vi "DaxKeyboardControl.vi"(8 "PlatMods":T1, 10 "Char":i16, 11 "Daxsonics Settings":refnum<vi>) -> ()   [LabVIEW 2022 SP3]
uses:
  Dax_Control_Cluster.ctl
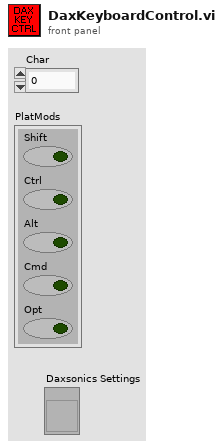
[diagram p1: front panel]
types:
  T1 = cluster{"Shift":bool, "Ctrl":bool, "Alt":bool, "Cmd":bool, "Opt":bool}
  T2 = typedef "Dax_Control_Cluster.ctl" = cluster{"Freq (MHz) ":u16, "Voltage (V)":u16, "Gain (dB)":u16}
  T3 = typedef "LVStringsAndValuesArrayTypeDef_U16.ctl" = cluster{"String":string, "Value":u16}[]
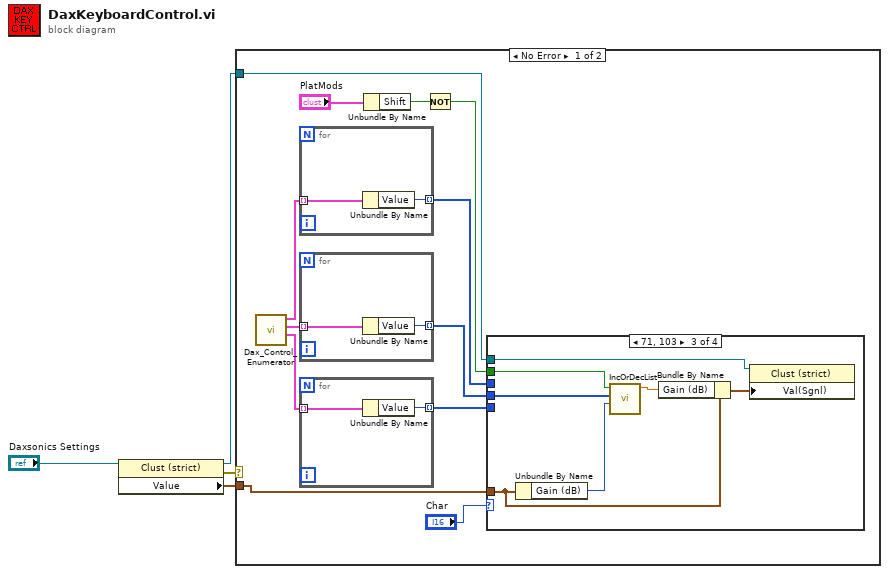
[diagram p0: block diagram]
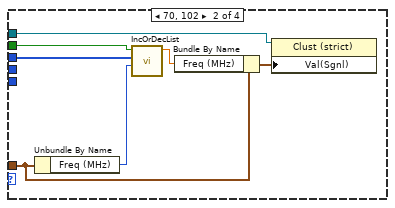
[diagram p3: hidden frame]
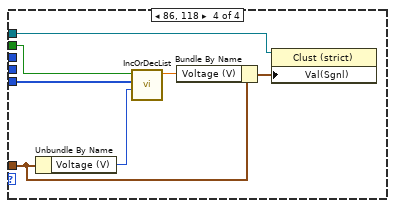
[diagram p4: hidden frame]
diagram:
  n1 = property on="Property Node" class="Clust (strict)"(reference="Daxsonics Settings") -> (reference out=w3:refnum<vi>, error out=w1:errorcluster, "Value"=w4:T2)  [unwired: 1 in]
  n2 = case shown="No Error" w1 {
    tunnel: w4 -> [w14 _]
    tunnel: w3 -> [w13 _]
    frame No Error {
      n3 = call "Dax_Control_Enumerator.vi"() -> ("Voltage"=w10:T3, "Gain"=w9:T3, "Freq"=w8:T3)  [unwired: 9 in]
      n4 = for {
        tunnel: w8 -> [w18] mode=indexing
        tunnel: [w17] -> w6 mode=indexing
        n5 = Unbundle By Name(w18) -> ("Value"=w17:u16)
      }
      n6 = for {
        tunnel: w9 -> [w20] mode=indexing
        tunnel: [w19] -> w7 mode=indexing
        n7 = Unbundle By Name(w20) -> ("Value"=w19:u16)
      }
      n8 = for {
        tunnel: w10 -> [w43] mode=indexing
        tunnel: [w42] -> w11 mode=indexing
        n9 = Unbundle By Name(w43) -> ("Value"=w42:u16)
      }
      n10 = Unbundle By Name("PlatMods") -> ("Shift"=w12:bool)
      n11 = Not(x=w12) -> (.not. x?=w5:bool)
      n12 = case shown="71, 103" "Char" {
        tunnel: w14 -> [_ w27 w34 w39]
        tunnel: w13 -> [_ w25 w32 w41]
        tunnel: w5 -> [_ w24 w31 w35]
        tunnel: w11 -> [_ _ _ w36]
        tunnel: w7 -> [_ _ w29 _]
        tunnel: w6 -> [_ w23 _ _]
        frame Default {
        }
        frame 70, 102 {
          n13 = Unbundle By Name(w27) -> ("Freq (MHz)"=w22:u16)
          n14 = call "IncOrDecList.vi"("Input"=w22, "Vals"=w23, "Shift"=w24) -> ("Output"=w21:dbl)  [unwired: 8 in]
          n15 = Bundle By Name(cluster=w27, "Freq (MHz)"=w21) -> (w26:T2)
          n16 = property class="Clust (strict)"(reference=w25, "Val(Sgnl)"=w26) -> ()  [unwired: 1 in, 2 out]
        }
        frame 71, 103 {
          n17 = Unbundle By Name(w34) -> ("Gain (dB)"=w28:u16)
          n18 = call "IncOrDecList.vi"("Input"=w28, "Vals"=w29, "Shift"=w31) -> ("Output"=w30:dbl)  [unwired: 8 in]
          n19 = Bundle By Name(cluster=w34, "Gain (dB)"=w30) -> (w33:T2)
          n20 = property class="Clust (strict)"(reference=w32, "Val(Sgnl)"=w33) -> ()  [unwired: 1 in, 2 out]
        }
        frame 86, 118 {
          n21 = Unbundle By Name(w39) -> ("Voltage (V)"=w38:u16)
          n22 = call "IncOrDecList.vi"("Input"=w38, "Vals"=w36, "Shift"=w35) -> ("Output"=w37:dbl)  [unwired: 8 in]
          n23 = Bundle By Name(cluster=w39, "Voltage (V)"=w37) -> (w40:T2)
          n24 = property class="Clust (strict)"(reference=w41, "Val(Sgnl)"=w40) -> ()  [unwired: 1 in, 2 out]
        }
      }
    }
    frame Error {
    }
  }
